vi "Stop RxTx.vi"(8 "error in (no error)":errorcluster, 11 "TCS in":refnum<class "TCS.lvclass">) -> (0 "error out":errorcluster, 3 "TCS out":refnum<class "TCS.lvclass">)   [LabVIEW 2018, in "TCS.lvclass"]
uses:
  TCS.lvclass
  TCS.lvclass/TCS.ctl
  RxTx/RxTx.lvclass
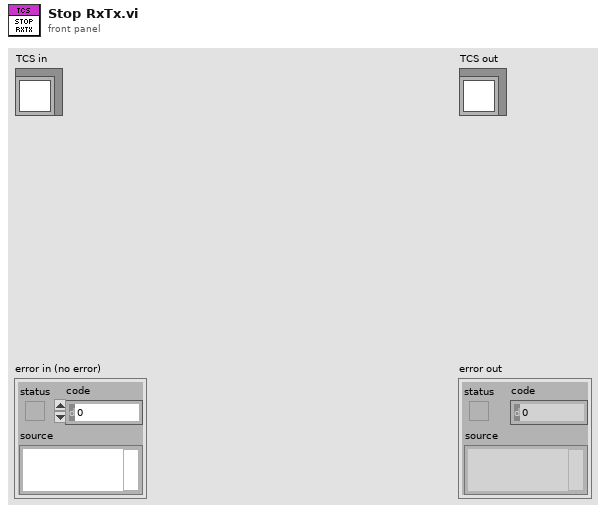
[diagram p1: front panel]
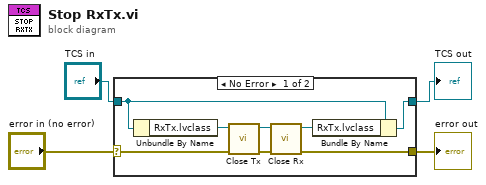
[diagram p0: block diagram]
diagram:
  n1 = case shown="No Error" "error in (no error)" {
    selector: "error in (no error)" -> [w8 w14]
    tunnel: [w5 w14] -> w3
    tunnel: [w11 w13] -> w1
    tunnel: "TCS in" -> [w12 w13]
    frame No Error {
      n2 = Unbundle By Name(w12) -> ("RxTx.lvclass"=w7:refnum<class "RxTx.lvclass">)
      n3 = call "Close Tx.vi"("error in (no error)"=w8, "RxTx in"=w7) -> ("error out"=w9:errorcluster, "RxTx out"=w10:refnum<class "RxTx.lvclass">)  [unwired: 8 in]
      n4 = call "Close Rx.vi"("error in (no error)"=w9, "RxTx in"=w10) -> ("error out"=w5:errorcluster, "RxTx out"=w6:refnum<class "RxTx.lvclass">)  [unwired: 8 in]
      n5 = Bundle By Name(cluster=w12, "RxTx.lvclass"=w6) -> (w11:refnum<class "TCS.lvclass">)
    }
    frame Error {
    }
  }
  "error out" <- w3
  "TCS out" <- w1
